vi "Log View for Frequency Response.vi"(2 "channel Y info":T1={"sensor sensitivity [mV/EU]"=1000.0, "engineering units"=1, "dB reference [EU]"=1.0, "custom label"="EU", "weighting filter"=0, "pregain [dB]"=0.0} {"pregain [dB]" format="%.2f"; "weighting filter" items=["Linear", "A-weighting", "B-weighting", "C-weighting", "ITU-R 468-4", "Dolby", "CCITT", "C-message"]; "dB reference [EU]" format="%^.1e"; "engineering units" items=["custom..."=0, "V"=1, "A"=21, "Pa"=2, "N"=20, "g"=3, "m/s^2"=4, "m/s"=5, "m"=6, "mm/s"=12, "mm"=13, "microns/s"=14, "microns"=15, "in/s^2"=7, "in/s"=8, "in"=9, "mils/s"=10, "mils"=11, "rad/s^2"=16, "rad/s"=17, "rad"=18, "strain"=19]; "sensor sensitivity [mV/EU]" format="%.2f"}, 3 "channel X info":T1={"sensor sensitivity [mV/EU]"=1000.0, "engineering units"=1, "dB reference [EU]"=1.0, "custom label"="EU", "weighting filter"=0, "pregain [dB]"=0.0} {"pregain [dB]" format="%.2f"; "weighting filter" items=["Linear", "A-weighting", "B-weighting", "C-weighting", "ITU-R 468-4", "Dolby", "CCITT", "C-message"]; "dB reference [EU]" format="%^.1e"; "engineering units" items=["custom..."=0, "V"=1, "A"=21, "Pa"=2, "N"=20, "g"=3, "m/s^2"=4, "m/s"=5, "m"=6, "mm/s"=12, "mm"=13, "microns/s"=14, "microns"=15, "in/s^2"=7, "in/s"=8, "in"=9, "mils/s"=10, "mils"=11, "rad/s^2"=16, "rad/s"=17, "rad"=18, "strain"=19]; "sensor sensitivity [mV/EU]" format="%.2f"}, 4 "dB On (T)":bool=TRUE, 5 "FRF [EUy/EUx]":dbl[](array[numeric]) format="%.2f") -> (0 "unit label":string, 1 "log view FRF [dB EUy/EUx]":dbl[](array[numeric]) format="%.2f")   [LabVIEW 2017]
uses:
  <vilib>/addons/Sound and Vibration/compatibility/Controls/svl_Channel Info.ctl
  <vilib>/addons/Sound and Vibration/compatibility/Controls/svl_Engineering Units Text Ring.ctl
  <vilib>/addons/Sound and Vibration/compatibility/Controls/svl_Weighting Filter Text Ring.ctl
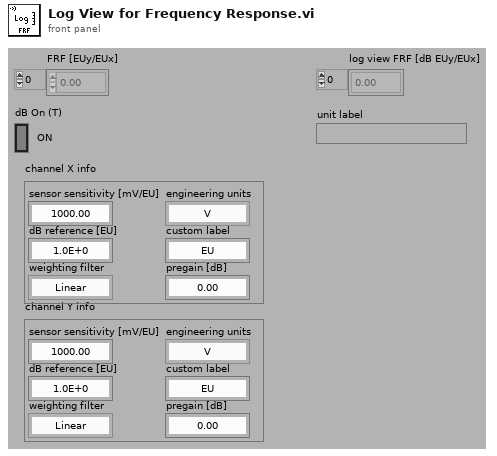
[diagram p1: front panel]
types:
  T1 = typedef "svl_Channel Info.ctl" = cluster{"sensor sensitivity [mV/EU]":dbl, "engineering units":T2, "dB reference [EU]":dbl, "custom label":string, "weighting filter":T3, "pregain [dB]":dbl}
  T2 = typedef "svl_Engineering Units Text Ring.ctl" = u16
  T3 = typedef "svl_Weighting Filter Text Ring.ctl" = u16
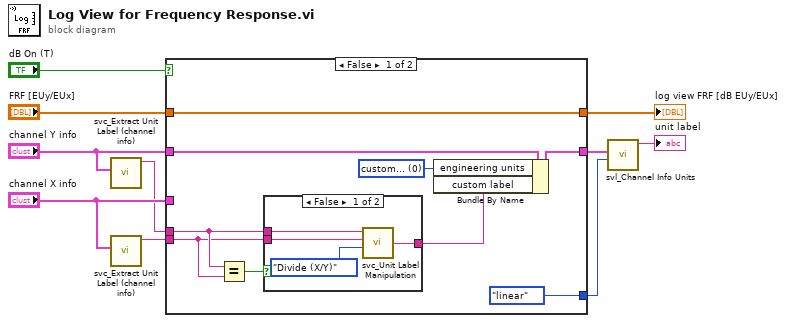
[diagram p0: block diagram]
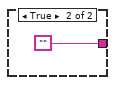
[diagram p2: hidden frame]
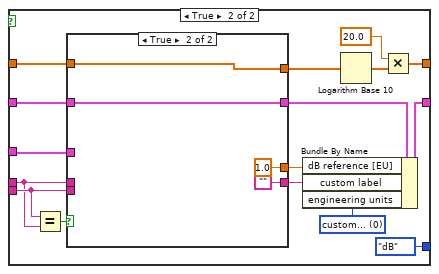
[diagram p3: hidden frame]
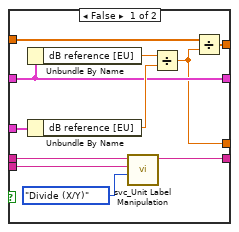
[diagram p4: hidden frame]
diagram:
  n1 = call <vilib>:"svc_Extract Unit Label (channel info).vi"("channel info"="channel Y info") -> ("unit label"=w4:string)  [unwired: 8 in, 2 out]
  n2 = call <vilib>:"svc_Extract Unit Label (channel info).vi"("channel info"="channel X info") -> ("unit label"=w5:string)  [unwired: 8 in, 2 out]
  n3 = case shown="False" "dB On (T)" {
    tunnel: [w16 w33] -> w8
    tunnel: "FRF [EUy/EUx]" -> [w16 w34]
    tunnel: w4 -> [w19 w37]
    tunnel: [w12 w29] -> w2
    tunnel: w5 -> [w18 w38]
    tunnel: "channel Y info" -> [w15 w40]
    tunnel: "channel X info" -> [_ w39]
    tunnel: [enum16{"linear", "dB"}."linear" ("linear/dB") enum16{"linear", "dB"}."dB" ("linear/dB")] -> w1
    frame False {
      w13 = u16 0 items=["custom...", "V", "Pa", "g", "m/s^2", "m/s", "m", "in/s^2", "in/s", "in", "mm", "mils", "A"] ("engineering units")
      n4 = Equal?(x=w19, y=w18) -> (x = y?=w17:bool)
      n5 = case shown="False" w17 {
        tunnel: [w23 ""] -> w14
        tunnel: w19 -> [w22 _]
        tunnel: w18 -> [w21 _]
        frame False {
          n6 = call <vilib>:"svc_Unit Label Manipulation.vi"("operation"=enum16{"Square (X^2)", "Divide (X/Y)"}."Divide (X/Y)", "Y unit label"=w21, "X unit label"=w22) -> ("resulting unit label"=w23:string)  [unwired: 4 in]
        }
        frame True {
        }
      }
      n7 = Bundle By Name(cluster=w15, "engineering units"=w13, "custom label"=w14) -> (w12:T1)
    }
    frame True {
      w27 = u16 0 items=["custom...", "V", "Pa", "g", "m/s^2", "m/s", "m", "in/s^2", "in/s", "in", "mm", "mils", "A"] ("engineering units")
      n8 = Equal?(x=w38, y=w37) -> (x = y?=w36:bool)
      n9 = case shown="True" w36 {
        tunnel: w40 -> [w43 w54]
        tunnel: w39 -> [w44 _]
        tunnel: w38 -> [w47 _]
        tunnel: w37 -> [w48 _]
        tunnel: [w46 w55] -> w35
        tunnel: w34 -> [w45 w55]
        tunnel: [w43 w54] -> w32
        tunnel: [w42 1.0] -> w28
        tunnel: [w41 ""] -> w26
        frame False {
          n10 = Unbundle By Name(w43) -> ("dB reference [EU]"=w51:dbl)
          n11 = Unbundle By Name(w44) -> ("dB reference [EU]"=w50:dbl)
          n12 = call <vilib>:"svc_Unit Label Manipulation.vi"("operation"=enum16{"Square (X^2)", "Divide (X/Y)"}."Divide (X/Y)", "Y unit label"=w47, "X unit label"=w48) -> ("resulting unit label"=w41:string)  [unwired: 4 in]
          n13 = Divide(x=w51, y=w50) -> (x/y=w42:dbl)
          n14 = Divide(x=w45, y=w42) -> (x/y=w46:dbl[])
        }
        frame True {
        }
      }
      n15 = Bundle By Name(cluster=w32, "dB reference [EU]"=w28, "custom label"=w26, "engineering units"=w27) -> (w29:T1)
      n16 = Logarithm Base 10(1:w35) -> (0:w30:dbl[])
      n17 = Multiply(x=20.0 ("y"), y=w30) -> (x*y=w33:dbl[])
    }
  }
  "log view FRF [dB EUy/EUx]" <- w8
  n18 = call <vilib>:"svl_Channel Info Units.vi"("linear/dB"=w1, "channel info"=w2) -> ("unit label"=→"unit label":string)  [unwired: 8 in, 1 out]
